vi "CRYpre-final Loudness.vi"(0 "Frame number":i32, 1 "Real matrix":dbl[][](array[numeric]), 5 "Version":i32, 7 "size":i32, 9 "Fe(stim)[n,kf]":T1=[[0.0, 0.0, 0.0, 0.0, 0.0, 0.0, 0.0, 0.0, 0.0, 0.0, 0.0, 0.0, 0.0, 0.0], [0.0, 0.0, 0.0, 40.0, 50.0, 80.0, 0.0, 0.0, 0.0, 0.0, 0.0, 0.0, 0.0, 0.0], [0.0, 0.0, 0.0, 60.0, 30.0, 0.0, 0.0, 0.0, 0.0, 0.0, 0.0, 0.0, 0.0, 0.0], [0.0, 0.0, 0.0, 0.0, 0.0, 0.0, 0.0, 0.0, 0.0, 0.0, 0.0, 0.0, 0.0, 0.0], [0.0, 0.0, 0.0, 0.0, 0.0, 0.0, 0.0, 0.0, 0.0, 0.0, 0.0, 0.0, 0.0, 0.0], [0.0, 0.0, 0.0, 0.0, 0.0, 0.0, 0.0, 0.0, 0.0, 0.0, 0.0, 0.0, 0.0, 0.0], [0.0, 0.0, 0.0, 0.0, 0.0, 0.0, 0.0, 0.0, 0.0, 0.0, 0.0, 0.0, 0.0, 0.0], [0.0, 0.0, 0.0, 0.0, 0.0, 0.0, 0.0, 0.0, 0.0, 0.0, 0.0, 0.0, 0.0, 0.0], [0.0, 0.0, 0.0, 0.0, 0.0, 0.0, 0.0, 0.0, 0.0, 0.0, 0.0, 0.0, 0.0, 0.0], [0.0, 0.0, 0.0, 0.0, 0.0, 0.0, 0.0, 0.0, 0.0, 0.0, 0.0, 0.0, 0.0, 0.0], [0.0, 0.0, 0.0, 0.0, 0.0, 0.0, 0.0, 0.0, 0.0, 0.0, 0.0, 0.0, 0.0, 0.0], [0.0, 0.0, 0.0, 0.0, 0.0, 0.0, 0.0, 0.0, 0.0, 0.0, 0.0, 0.0, 0.0, 0.0], [0.0, 0.0, 0.0, 0.0, 0.0, 0.0, 0.0, 0.0, 0.0, 0.0, 0.0, 0.0, 0.0, 0.0], [0.0, 0.0, 0.0, 0.0, 0.0, 0.0, 0.0, 0.0, 0.0, 0.0, 0.0, 0.0, 0.0, 0.0], [0.0, 0.0, 0.0, 0.0, 0.0, 0.0, 0.0, 0.0, 0.0, 0.0, 0.0, 0.0, 0.0, 0.0], [0.0, 0.0, 0.0, 0.0, 0.0, 0.0, 0.0, 0.0, 0.0, 0.0, 0.0, 0.0, 0.0, 0.0], [0.0, 0.0, 0.0, 0.0, 0.0, 0.0, 0.0, 0.0, 0.0, 0.0, 0.0, 0.0, 0.0, 0.0], [0.0, 0.0, 0.0, 0.0, 0.0, 0.0, 0.0, 0.0, 0.0, 0.0, 0.0, 0.0, 0.0, 0.0], [0.0, 0.0, 0.0, 0.0, 0.0, 0.0, 0.0, 0.0, 0.0, 0.0, 0.0, 0.0, 0.0, 0.0], [0.0, 0.0, 0.0, 0.0, 0.0, 0.0, 0.0, 0.0, 0.0, 0.0, 0.0, 0.0, 0.0, 0.0], [0.0, 0.0, 0.0, 0.0, 0.0, 0.0, 0.0, 0.0, 0.0, 0.0, 0.0, 0.0, 0.0, 0.0], [0.0, 0.0, 0.0, 0.0, 0.0, 0.0, 0.0, 0.0, 0.0, 0.0, 0.0, 0.0, 0.0, 0.0], [0.0, 0.0, 0.0, 0.0, 0.0, 0.0, 0.0, 0.0, 0.0, 0.0, 0.0, 0.0, 0.0, 0.0], [0.0, 0.0, 0.0, 0.0, 0.0, 0.0, 0.0, 0.0, 0.0, 0.0, 0.0, 0.0, 0.0, 0.0], [0.0, 0.0, 0.0, 0.0, 0.0, 0.0, 0.0, 0.0, 0.0, 0.0, 0.0, 0.0, 0.0, 0.0], [0.0, 0.0, 0.0, 0.0, 0.0, 0.0, 0.0, 0.0, 0.0, 0.0, 0.0, 0.0, 0.0, 0.0], [0.0, 0.0, 0.0, 0.0, 0.0, 0.0, 0.0, 0.0, 0.0, 0.0, 0.0, 0.0, 0.0, 0.0], [0.0, 0.0, 0.0, 0.0, 0.0, 0.0, 0.0, 0.0, 0.0, 0.0, 0.0, 0.0, 0.0, 0.0], [0.0, 0.0, 0.0, 0.0, 0.0, 0.0, 0.0, 0.0, 0.0, 0.0, 0.0, 0.0, 0.0, 0.0], [0.0, 0.0, 0.0, 0.0, 0.0, 0.0, 0.0, 0.0, 0.0, 0.0, 0.0, 0.0, 0.0, 0.0], [0.0, 0.0, 0.0, 0.0, 0.0, 0.0, 0.0, 0.0, 0.0, 0.0, 0.0, 0.0, 0.0, 0.0], [0.0, 0.0, 0.0, 0.0, 0.0, 0.0, 0.0, 0.0, 0.0, 0.0, 0.0, 0.0, 0.0, 0.0], [0.0, 0.0, 0.0, 0.0, 0.0, 0.0, 0.0, 0.0, 0.0, 0.0, 0.0, 0.0, 0.0, 0.0], [0.0, 0.0, 0.0, 0.0, 0.0, 0.0, 0.0, 0.0, 0.0, 0.0, 0.0, 0.0, 0.0, 0.0], [0.0, 0.0, 0.0, 0.0, 0.0, 0.0, 0.0, 0.0, 0.0, 0.0, 0.0, 0.0, 0.0, 0.0], [0.0, 0.0, 0.0, 0.0, 0.0, 0.0, 0.0, 0.0, 0.0, 0.0, 0.0, 0.0, 0.0, 0.0], [0.0, 0.0, 0.0, 0.0, 0.0, 0.0, 0.0, 0.0, 0.0, 0.0, 0.0, 0.0, 0.0, 0.0], [0.0, 0.0, 0.0, 0.0, 0.0, 0.0, 0.0, 0.0, 0.0, 0.0, 0.0, 0.0, 0.0, 0.0], [0.0, 0.0, 0.0, 0.0, 0.0, 0.0, 0.0, 0.0, 0.0, 0.0, 0.0, 0.0, 0.0, 0.0], [0.0, 0.0, 0.0, 0.0, 0.0, 0.0, 0.0, 0.0, 0.0, 0.0, 0.0, 0.0, 0.0, 0.0], [0.0, 0.0, 0.0, 0.0, 0.0, 0.0, 0.0, 0.0, 0.0, 0.0, 0.0, 0.0, 0.0, 22.0]], 11 "Fe(res)[n,kf]":T1=[[0.0, 0.0, 0.0, 0.0, 0.0, 0.0, 0.0, 0.0, 0.0, 0.0, 0.0, 0.0, 0.0, 0.0], [0.0, 0.0, 0.0, 40.0, 50.0, 80.0, 0.0, 0.0, 0.0, 0.0, 0.0, 0.0, 0.0, 0.0], [0.0, 0.0, 0.0, 60.0, 30.0, 0.0, 0.0, 0.0, 0.0, 0.0, 0.0, 0.0, 0.0, 0.0], [0.0, 0.0, 0.0, 0.0, 0.0, 0.0, 0.0, 0.0, 0.0, 0.0, 0.0, 0.0, 0.0, 0.0], [0.0, 0.0, 0.0, 0.0, 0.0, 0.0, 0.0, 0.0, 0.0, 0.0, 0.0, 0.0, 0.0, 0.0], [0.0, 0.0, 0.0, 0.0, 0.0, 0.0, 0.0, 0.0, 0.0, 0.0, 0.0, 0.0, 0.0, 0.0], [0.0, 0.0, 0.0, 0.0, 0.0, 0.0, 0.0, 0.0, 0.0, 0.0, 0.0, 0.0, 0.0, 0.0], [0.0, 0.0, 0.0, 0.0, 0.0, 0.0, 0.0, 0.0, 0.0, 0.0, 0.0, 0.0, 0.0, 0.0], [0.0, 0.0, 0.0, 0.0, 0.0, 0.0, 0.0, 0.0, 0.0, 0.0, 0.0, 0.0, 0.0, 0.0], [0.0, 0.0, 0.0, 0.0, 0.0, 0.0, 0.0, 0.0, 0.0, 0.0, 0.0, 0.0, 0.0, 0.0], [0.0, 0.0, 0.0, 0.0, 0.0, 0.0, 0.0, 0.0, 0.0, 0.0, 0.0, 0.0, 0.0, 0.0], [0.0, 0.0, 0.0, 0.0, 0.0, 0.0, 0.0, 0.0, 0.0, 0.0, 0.0, 0.0, 0.0, 0.0], [0.0, 0.0, 0.0, 0.0, 0.0, 0.0, 0.0, 0.0, 0.0, 0.0, 0.0, 0.0, 0.0, 0.0], [0.0, 0.0, 0.0, 0.0, 0.0, 0.0, 0.0, 0.0, 0.0, 0.0, 0.0, 0.0, 0.0, 0.0], [0.0, 0.0, 0.0, 0.0, 0.0, 0.0, 0.0, 0.0, 0.0, 0.0, 0.0, 0.0, 0.0, 0.0], [0.0, 0.0, 0.0, 0.0, 0.0, 0.0, 0.0, 0.0, 0.0, 0.0, 0.0, 0.0, 0.0, 0.0], [0.0, 0.0, 0.0, 0.0, 0.0, 0.0, 0.0, 0.0, 0.0, 0.0, 0.0, 0.0, 0.0, 0.0], [0.0, 0.0, 0.0, 0.0, 0.0, 0.0, 0.0, 0.0, 0.0, 0.0, 0.0, 0.0, 0.0, 0.0], [0.0, 0.0, 0.0, 0.0, 0.0, 0.0, 0.0, 0.0, 0.0, 0.0, 0.0, 0.0, 0.0, 0.0], [0.0, 0.0, 0.0, 0.0, 0.0, 0.0, 0.0, 0.0, 0.0, 0.0, 0.0, 0.0, 0.0, 0.0], [0.0, 0.0, 0.0, 0.0, 0.0, 0.0, 0.0, 0.0, 0.0, 0.0, 0.0, 0.0, 0.0, 0.0], [0.0, 0.0, 0.0, 0.0, 0.0, 0.0, 0.0, 0.0, 0.0, 0.0, 0.0, 0.0, 0.0, 0.0], [0.0, 0.0, 0.0, 0.0, 0.0, 0.0, 0.0, 0.0, 0.0, 0.0, 0.0, 0.0, 0.0, 0.0], [0.0, 0.0, 0.0, 0.0, 0.0, 0.0, 0.0, 0.0, 0.0, 0.0, 0.0, 0.0, 0.0, 0.0], [0.0, 0.0, 0.0, 0.0, 0.0, 0.0, 0.0, 0.0, 0.0, 0.0, 0.0, 0.0, 0.0, 0.0], [0.0, 0.0, 0.0, 0.0, 0.0, 0.0, 0.0, 0.0, 0.0, 0.0, 0.0, 0.0, 0.0, 0.0], [0.0, 0.0, 0.0, 0.0, 0.0, 0.0, 0.0, 0.0, 0.0, 0.0, 0.0, 0.0, 0.0, 0.0], [0.0, 0.0, 0.0, 0.0, 0.0, 0.0, 0.0, 0.0, 0.0, 0.0, 0.0, 0.0, 0.0, 0.0], [0.0, 0.0, 0.0, 0.0, 0.0, 0.0, 0.0, 0.0, 0.0, 0.0, 0.0, 0.0, 0.0, 0.0], [0.0, 0.0, 0.0, 0.0, 0.0, 0.0, 0.0, 0.0, 0.0, 0.0, 0.0, 0.0, 0.0, 0.0], [0.0, 0.0, 0.0, 0.0, 0.0, 0.0, 0.0, 0.0, 0.0, 0.0, 0.0, 0.0, 0.0, 0.0], [0.0, 0.0, 0.0, 0.0, 0.0, 0.0, 0.0, 0.0, 0.0, 0.0, 0.0, 0.0, 0.0, 0.0], [0.0, 0.0, 0.0, 0.0, 0.0, 0.0, 0.0, 0.0, 0.0, 0.0, 0.0, 0.0, 0.0, 0.0], [0.0, 0.0, 0.0, 0.0, 0.0, 0.0, 0.0, 0.0, 0.0, 0.0, 0.0, 0.0, 0.0, 0.0], [0.0, 0.0, 0.0, 0.0, 0.0, 0.0, 0.0, 0.0, 0.0, 0.0, 0.0, 0.0, 0.0, 0.0], [0.0, 0.0, 0.0, 0.0, 0.0, 0.0, 0.0, 0.0, 0.0, 0.0, 0.0, 0.0, 0.0, 0.0], [0.0, 0.0, 0.0, 0.0, 0.0, 0.0, 0.0, 0.0, 0.0, 0.0, 0.0, 0.0, 0.0, 0.0], [0.0, 0.0, 0.0, 0.0, 0.0, 0.0, 0.0, 0.0, 0.0, 0.0, 0.0, 0.0, 0.0, 0.0], [0.0, 0.0, 0.0, 0.0, 0.0, 0.0, 0.0, 0.0, 0.0, 0.0, 0.0, 0.0, 0.0, 0.0], [0.0, 0.0, 0.0, 0.0, 0.0, 0.0, 0.0, 0.0, 0.0, 0.0, 0.0, 0.0, 0.0, 0.0], [0.0, 0.0, 0.0, 0.0, 0.0, 0.0, 0.0, 0.0, 0.0, 0.0, 0.0, 0.0, 0.0, 22.0]]) -> (4 "total Loudness":dbl)   [LabVIEW 2013]
uses:
  <vilib>/Analysis/Matrix/Datatypes/RealMatrix.ctl
  <vilib>/Analysis/Matrix/NI_Matrix.lvlib
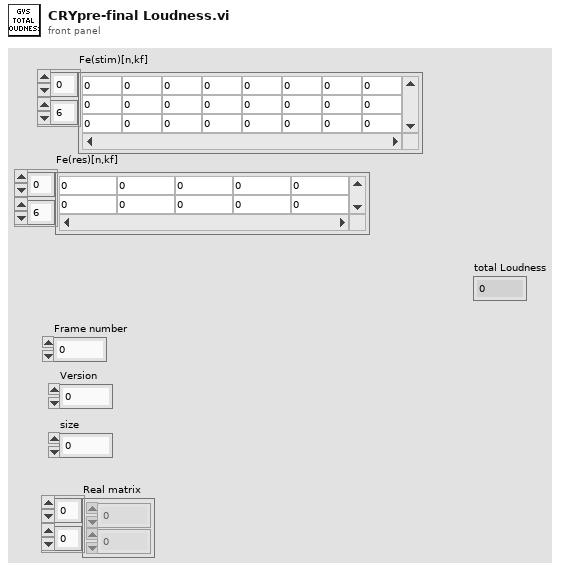
[diagram p1: front panel]
types:
  T1 = typedef "NI_Matrix.lvlib/RealMatrix.ctl" = dbl[][]
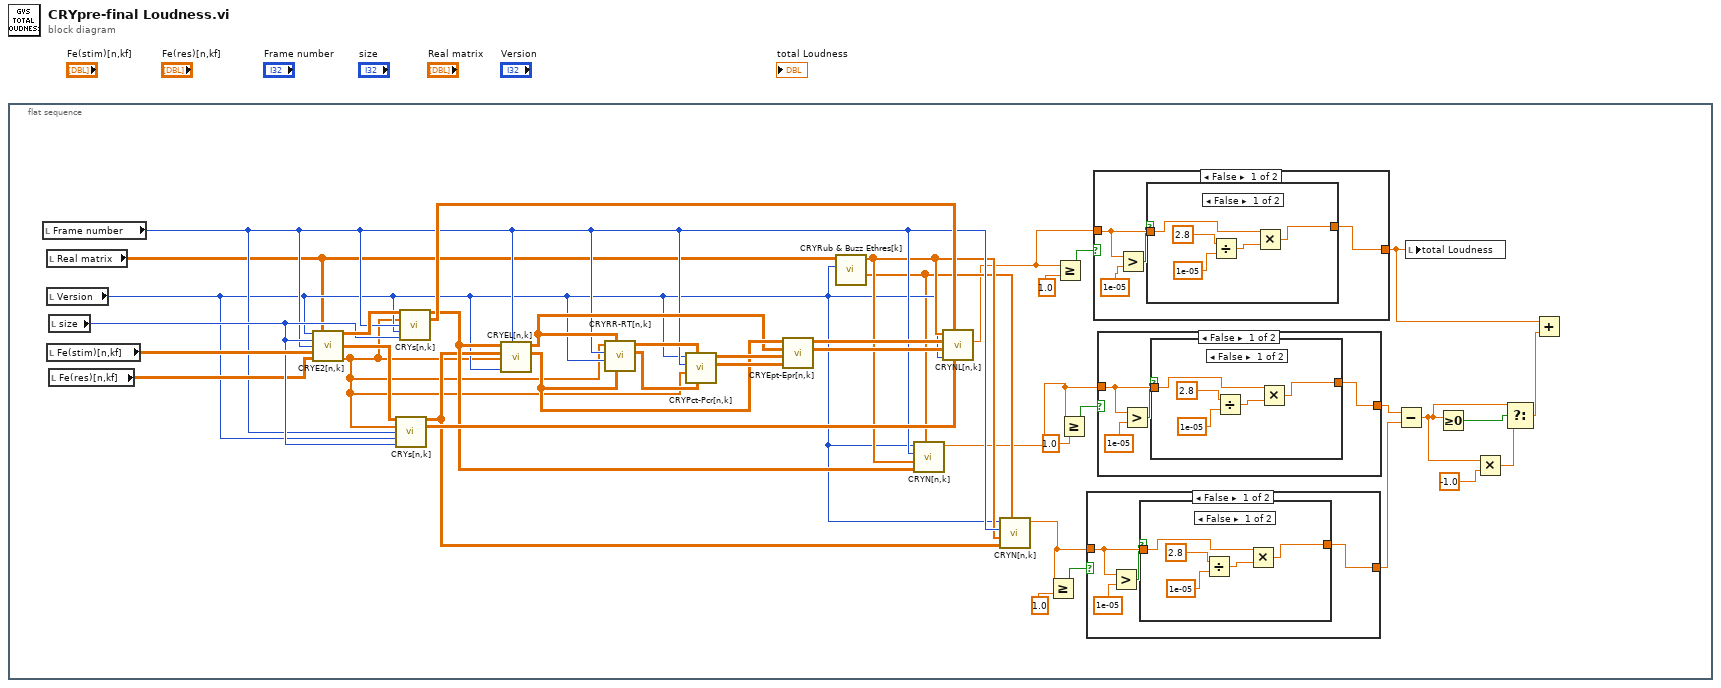
[diagram p0: block diagram]
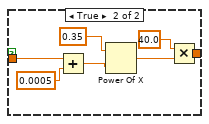
[diagram p2: hidden frame]
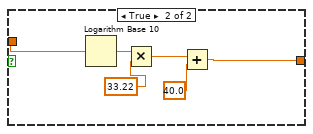
[diagram p3: hidden frame]
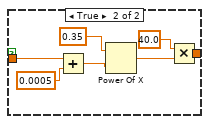
[diagram p4: hidden frame]
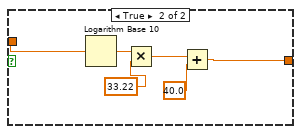
[diagram p5: hidden frame]
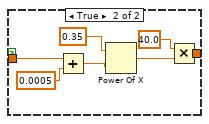
[diagram p6: hidden frame]
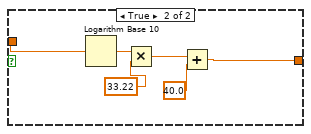
[diagram p7: hidden frame]
diagram:
  n1 = flat-sequence {
    frame #0 {
      n2 = local read "Frame number"() -> (w23:i32)
      n3 = local read "Real matrix"() -> (w18:dbl[][])
      n4 = local read "Version"() -> (w21:i32)
      n5 = local read "Fe(stim)[n,kf]"() -> (w30:T1)
      n6 = local read "size"() -> (w29:i32)
      n7 = local read "Fe(res)[n,kf]"() -> (w28:T1)
      n8 = call "CRYE2[n,k].vi"("Version"=w21, "Real matrix"=w18, "size"=w29, "Frame number"=w23, "Fe(stim)[n,kf]"=w30, "Fe(res)[n,kf]"=w28) -> ("E2(stim)[n,kf]"=w40:T1, "E2(res)[n,kf]"=w39:T1, "alfa[k]"=w19:dbl[])  [unwired: 7 in]
      n9 = call "CRYs[n,k].vi"("E2[n,kf]"=w39, "alfa[k]"=w19, "Frame number"=w23, "Version"=w21, "size"=w29) -> ("E[n,kf]"=w24:T1, "s[n,kf]"=w33:T1)  [unwired: 9 in]
      n10 = call "CRYs[n,k].vi"("E2[n,kf]"=w40, "alfa[k]"=w19, "Frame number"=w23, "Version"=w21, "size"=w29) -> ("E[n,kf]"=w25:T1, "s[n,kf]"=w34:T1)  [unwired: 9 in]
      n11 = call "CRYEL[n,k].vi"("Frame number"=w23, "Version"=w21, "alfa[k]"=w19, "E(res)[n,kf]"=w24, "E(stim)[n,kf]"=w25) -> ("EL(res)[n,kf]"=w27:T1, "EL(stim)[n,kf]"=w26:T1)  [unwired: 4 in, 1 out]
      n12 = call "CRYRR-RT[n,k].vi"("EL(res)[n,kf]"=w27, "EL(stim)[n,kf]"=w26, "Version"=w21, "Frame number"=w23, "alfa[k]"=w19) -> ("RR(stim)[n,kf]"=w37:T1, "RT(res)[n,kf]"=w38:T1)  [unwired: 5 in]
      n13 = call "CRYPct-Pcr[n,k].vi"("RR(stim)[n,kf]"=w37, "RT(res)[n,kf]"=w38, "alfa[k]"=w19, "Frame number"=w23, "Version"=w21) -> ("Pcr[n,kf]"=w35:T1, "Pct[n,kf]"=w36:T1)  [unwired: 5 in]
      n14 = call "CRYEpt-Epr[n,k].vi"("ELT(res)[n,kf]"=w27, "ELR(stim)[n,kf]"=w26, "Pct[n,kf]"=w36, "Pcr[n,kf]"=w35) -> ("Ept(res)[n,kf]"=w32:T1, "Epr(stim)[n,kf]"=w31:T1)  [unwired: 4 in]
      n15 = call "CRYRub & Buzz Ethres[k].vi"("Version"=w21, "Real matrix"=w18) -> ("s[k]"=w20:dbl[], "Ethres[k]"=w22:dbl[])  [unwired: 7 in]
      n16 = call "CRYN[n,k].vi"("s[k]"=w20, "E[n,kf]"=w25, "Ethres[k]"=w22, "Frame number"=w23, "Version"=w21) -> ("total Loudness"=w7:dbl)  [unwired: 6 in]
      n17 = call "CRYNL[n,k].vi"("sr(stim)[n,kf]"=w33, "st(res)[n,kf]"=w34, "Version"=w21, "Epr(stim)[n,kf]"=w31, "Ept(res)[n,kf]"=w32, "Ethres[k]"=w22) -> ("total Loudness"=w3:dbl)  [unwired: 3 in, 1 out]
      n18 = call "CRYN[n,k].vi"("s[k]"=w20, "E[n,kf]"=w24, "Ethres[k]"=w22, "Frame number"=w23, "Version"=w21) -> ("total Loudness"=w10:dbl)  [unwired: 6 in]
      n19 = Greater Or Equal?(x=w10, y=1.0) -> (x >= y?=w11:bool)
      n20 = Greater Or Equal?(x=w3, y=1.0) -> (x >= y?=w4:bool)
      n21 = Greater Or Equal?(x=w7, y=1.0) -> (x >= y?=w8:bool)
      n22 = case shown="False" w11 {
        tunnel: w10 -> [w86 w106]
        tunnel: [w88 w101] -> w9
        frame False {
          n23 = Greater?(x=w86, y=1e-05) -> (0:w85:bool)
          n24 = case shown="False" w85 {
            tunnel: [w89 w95] -> w88
            tunnel: w86 -> [w90 w94]
            frame False {
              n25 = Divide(x=2.8, y=1e-05) -> (x/y=w91:dbl)
              n26 = Multiply(x=w90, y=w91) -> (x*y=w89:dbl)
            }
            frame True {
              n27 = Add(x=w94, y=0.0005) -> (x+y=w99:dbl)
              n28 = Power Of X(1:w99, 2:0.35) -> (0:w97:dbl)
              n29 = Multiply(x=40.0, y=w97) -> (x*y=w95:dbl)
            }
          }
        }
        frame True {
          n30 = Logarithm Base 10(1:w106) -> (0:w105:dbl)
          n31 = Multiply(x=w105, y=33.22) -> (x*y=w103:dbl)
          n32 = Add(x=w103, y=40.0) -> (x+y=w101:dbl)
        }
      }
      n33 = case shown="False" w4 {
        tunnel: w3 -> [w42 w62]
        tunnel: [w44 w57] -> w2
        frame False {
          n34 = Greater?(x=w42, y=1e-05) -> (0:w41:bool)
          n35 = case shown="False" w41 {
            tunnel: [w45 w51] -> w44
            tunnel: w42 -> [w46 w50]
            frame False {
              n36 = Divide(x=2.8, y=1e-05) -> (x/y=w47:dbl)
              n37 = Multiply(x=w46, y=w47) -> (x*y=w45:dbl)
            }
            frame True {
              n38 = Add(x=w50, y=0.0005) -> (x+y=w55:dbl)
              n39 = Power Of X(1:w55, 2:0.35) -> (0:w53:dbl)
              n40 = Multiply(x=40.0, y=w53) -> (x*y=w51:dbl)
            }
          }
        }
        frame True {
          n41 = Logarithm Base 10(1:w62) -> (0:w61:dbl)
          n42 = Multiply(x=w61, y=33.22) -> (x*y=w59:dbl)
          n43 = Add(x=w59, y=40.0) -> (x+y=w57:dbl)
        }
      }
      n44 = case shown="False" w8 {
        tunnel: w7 -> [w64 w84]
        tunnel: [w66 w79] -> w6
        frame False {
          n45 = Greater?(x=w64, y=1e-05) -> (0:w63:bool)
          n46 = case shown="False" w63 {
            tunnel: [w67 w73] -> w66
            tunnel: w64 -> [w68 w72]
            frame False {
              n47 = Divide(x=2.8, y=1e-05) -> (x/y=w69:dbl)
              n48 = Multiply(x=w68, y=w69) -> (x*y=w67:dbl)
            }
            frame True {
              n49 = Add(x=w72, y=0.0005) -> (x+y=w77:dbl)
              n50 = Power Of X(1:w77, 2:0.35) -> (0:w75:dbl)
              n51 = Multiply(x=40.0, y=w75) -> (x*y=w73:dbl)
            }
          }
        }
        frame True {
          n52 = Logarithm Base 10(1:w84) -> (0:w83:dbl)
          n53 = Multiply(x=w83, y=33.22) -> (x*y=w81:dbl)
          n54 = Add(x=w81, y=40.0) -> (x+y=w79:dbl)
        }
      }
      n55 = Subtract(x=w6, y=w9) -> (x-y=w15:dbl)
      n56 = local write "total Loudness"(w2) -> ()
      n57 = Greater Or Equal To 0?(x=w15) -> (x >= 0?=w17:bool)
      n58 = Multiply(x=w15, y=-1.0) -> (x*y=w14:dbl)
      n59 = Select(t=w15, s=w17, f=w14) -> (s? t:f=w13:dbl)
      n60 = Add(x=w2, y=w13) -> ()  [unwired: 1 out]
    }
  }
